vi "PG-filter.vi"(10 "Y":dbl[](array[numeric]), 11 "n":i16) -> (3 "数组":ext[](array[numeric]))   [LabVIEW 2014]
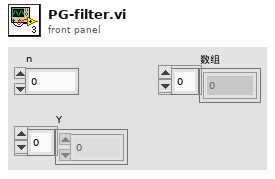
[diagram p1: front panel]
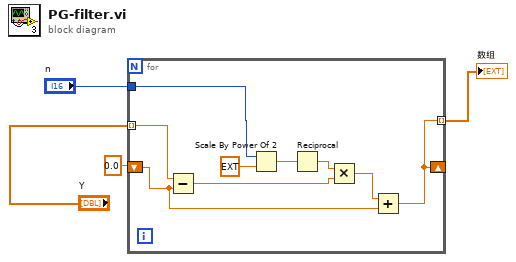
[diagram p0: block diagram]
diagram:
  n1 = for {
    shift-right: [w6] -> _
    shift-left: 0.0 -> [w7]
    tunnel: "Y" -> [w10] mode=indexing
    tunnel: [w6] -> w2 mode=indexing
    tunnel: "n" -> [w5]
    n2 = Subtract(x=w10, y=w7) -> (x-y=w9:ext)
    n3 = Scale By Power Of 2(n=w5, x=ext 1.0) -> (x*2^n=w12:ext)
    n4 = Reciprocal(x=w12) -> (1/x=w11:ext)
    n5 = Multiply(x=w11, y=w9) -> (x*y=w8:ext)
    n6 = Add(x=w8, y=w7) -> (x+y=w6:ext)
  }
  "数组" <- w2
